vi "Convert Data to Gain values.vi"(0 "Messages":T1(array[cluster])) -> (14 "Gain A":sgl, 15 "Gain B":sgl, 16 "Gain C":sgl)   [LabVIEW 2023]
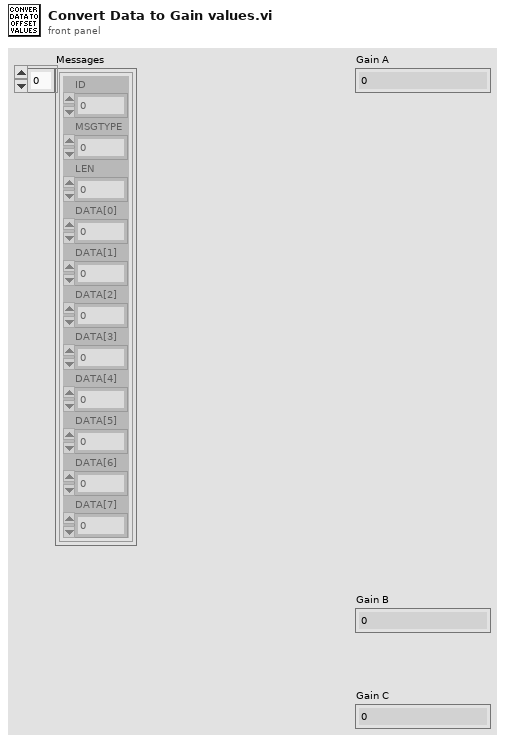
[diagram p1: front panel]
types:
  T1 = cluster{"ID":u32, "MSGTYPE":u8, "LEN":u8, "DATA[0]":u8, "DATA[1]":u8, "DATA[2]":u8, "DATA[3]":u8, "DATA[4]":u8, "DATA[5]":u8, "DATA[6]":u8, "DATA[7]":u8}[]
  T2 = cluster{"ID":u32, "MSGTYPE":u8, "LEN":u8, "DATA[0]":u8, "DATA[1]":u8, "DATA[2]":u8, "DATA[3]":u8, "DATA[4]":u8, "DATA[5]":u8, "DATA[6]":u8, "DATA[7]":u8}
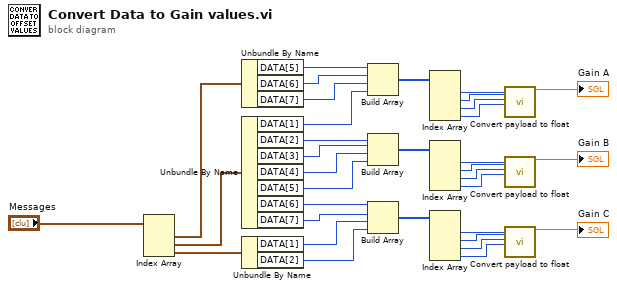
[diagram p0: block diagram]
diagram:
  n1 = Index Array(array="Messages") -> (element #1=w33:T2, element #2=w32:T2, element #3=w31:T2)  [unwired: 3 in]
  n2 = Unbundle By Name(w33) -> ("DATA[5]"=w30:u8, "DATA[6]"=w29:u8, "DATA[7]"=w28:u8)
  n3 = Unbundle By Name(w32) -> ("DATA[1]"=w27:u8, "DATA[2]"=w26:u8, "DATA[3]"=w25:u8, "DATA[4]"=w24:u8, "DATA[5]"=w23:u8, "DATA[6]"=w22:u8, "DATA[7]"=w21:u8)
  n4 = Unbundle By Name(w31) -> ("DATA[1]"=w20:u8, "DATA[2]"=w19:u8)
  n5 = Build Array(w30, w29, w28, w27) -> (w18:u8[])
  n6 = Build Array(w26, w25, w24, w23) -> (w8:u8[])
  n7 = Build Array(w22, w21, w20, w19) -> (w3:u8[])
  n8 = Index Array(array=w18) -> (element #1=w17:u8, element #2=w16:u8, element #3=w15:u8, element #4=w14:u8)  [unwired: 4 in]
  n9 = Index Array(array=w8) -> (element #1=w9:u8, element #2=w10:u8, element #3=w11:u8, element #4=w12:u8)  [unwired: 4 in]
  n10 = Index Array(array=w3) -> (element #1=w7:u8, element #2=w6:u8, element #3=w5:u8, element #4=w4:u8)  [unwired: 4 in]
  n11 = call "Convert payload to float.vi"("Byte1"=w17, "Byte2"=w16, "Byte3"=w15, "Byte4"=w14) -> ("FloatNumber"=→"Gain A":sgl)  [unwired: 15 in]
  n12 = call "Convert payload to float.vi"("Byte1"=w9, "Byte2"=w10, "Byte3"=w11, "Byte4"=w12) -> ("FloatNumber"=→"Gain B":sgl)  [unwired: 15 in]
  n13 = call "Convert payload to float.vi"("Byte1"=w7, "Byte2"=w6, "Byte3"=w5, "Byte4"=w4) -> ("FloatNumber"=→"Gain C":sgl)  [unwired: 15 in]
